vi "WPI_RelaySetArraysInCache.vi"(0 "Relay Direction":T2, 1 "forward array  in":bool[](array[boolean]), 2 "reverse array in":bool[](array[boolean]), 3 "array index":T1=enum."Relay 1", 4 "new value":bool) -> (5 "forward array out":bool[](array[boolean]), 6 "reverse array out":bool[](array[boolean]))   [LabVIEW 2017]
doc: "This software is licensed. Open the labview\\readme\\WPI Robotics Library Open Source License.txt file for more information."
uses:
  <vilib>/Rock Robotics/WPI/Relay/WPI_RelayDirection.ctl
  <vilib>/Rock Robotics/SystemInterfaces/DIO/FPGA_DIORelayChannel.ctl
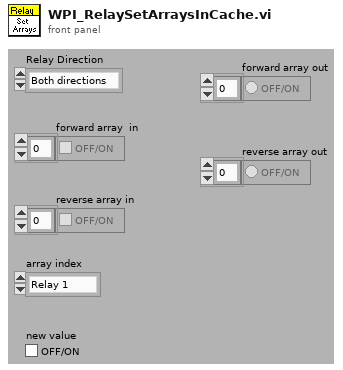
[diagram p1: front panel]
types:
  T1 = typedef "FPGA_DIORelayChannel.ctl" = enum8{"Relay 0", "Relay 1", "Relay 2", "Relay 3", "Invalid"}
  T2 = typedef "WPI_RelayDirection.ctl" = enum16{"Both directions", "Forward only", "Reverse only"}
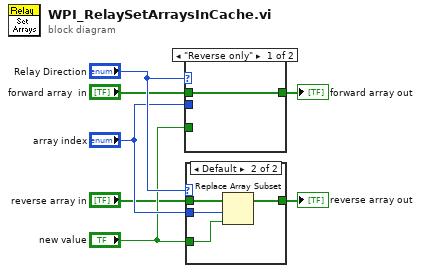
[diagram p0: block diagram]
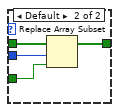
[diagram p2: hidden frame]
diagram:
  n1 = case shown="\"Reverse only\"" "Relay Direction" {
    tunnel: "new value" -> [_ w12]
    tunnel: "forward array  in" -> [w8 w11]
    tunnel: [w8 w10] -> w6
    tunnel: "array index" -> [_ w9]
    frame "Reverse only" {
    }
    frame Default {
      n2 = Replace Array Subset(array=w11, new element=w12, index=w9) -> (w10:bool[])
    }
  }
  "forward array out" <- w6
  n3 = case shown="Default" "Relay Direction" {
    tunnel: "new value" -> [_ w17]
    tunnel: "reverse array in" -> [w13 w16]
    tunnel: [w13 w15] -> w2
    tunnel: "array index" -> [_ w14]
    frame "Forward only" {
    }
    frame Default {
      n4 = Replace Array Subset(array=w16, new element=w17, index=w14) -> (w15:bool[])
    }
  }
  "reverse array out" <- w2
